vi "IQ Inversion.vi"(0 "input data":T1[](array[typedef])=[{"I"=0.0, "Q"=0.0, "overflow"=FALSE}, {"I"=0.0, "Q"=0.0, "overflow"=FALSE}, {"I"=0.0, "Q"=0.0, "overflow"=FALSE}, {"I"=0.0, "Q"=0.0, "overflow"=FALSE}, {"I"=0.0, "Q"=0.0, "overflow"=FALSE}, {"I"=0.0, "Q"=0.0, "overflow"=FALSE}, {"I"=0.0, "Q"=0.0, "overflow"=FALSE}, {"I"=0.0, "Q"=0.0, "overflow"=FALSE}, {"I"=0.0, "Q"=0.0, "overflow"=FALSE}, {"I"=0.0, "Q"=0.0, "overflow"=FALSE}, {"I"=0.0, "Q"=0.0, "overflow"=FALSE}, {"I"=0.0, "Q"=0.0, "overflow"=FALSE}, {"I"=0.0, "Q"=0.0, "overflow"=FALSE}, {"I"=0.0, "Q"=0.0, "overflow"=FALSE}, {"I"=0.0, "Q"=0.0, "overflow"=FALSE}, {"I"=0.0, "Q"=0.0, "overflow"=FALSE}], 5 "IQ inversion":cluster{"invert I":bool, "invert Q":bool}, 9 "input valid":bool=TRUE) -> (4 "output data":T1[](array[typedef]), 10 "output valid":bool)   [LabVIEW 2019]
uses:
  <instrlib>/_niInstr/DSP/v1/Shared/Public/IQ Data.ctl
  <instrlib>/_niInstr/DSP/v1/Shared/niInstr DSP v1 Shared.lvlib
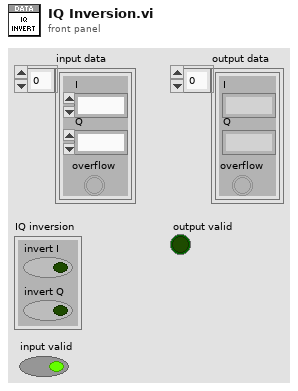
[diagram p1: front panel]
types:
  T1 = typedef "niInstr DSP v1 Shared.lvlib/IQ Data.ctl" = cluster{"I":fxp<+/-,18,1>, "Q":fxp<+/-,18,1>, "overflow":bool}
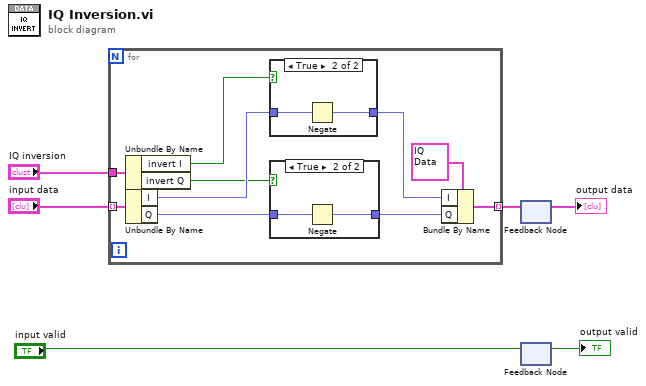
[diagram p0: block diagram]
diagram:
  n1 = for {
    tunnel: "input data" -> [w16] mode=indexing
    tunnel: "IQ inversion" -> [w15]
    tunnel: [w8] -> w4 mode=indexing
    n2 = Unbundle By Name(w15) -> ("invert I"=w14:bool, "invert Q"=w12:bool)
    n3 = Unbundle By Name(w16) -> ("I"=w13:fxp<+/-,18,1>, "Q"=w11:fxp<+/-,18,1>)
    n4 = case shown="True" w14 {
      tunnel: w13 -> [w20 w22]
      tunnel: [w20 w21] -> w10
      frame False {
      }
      frame True {
        n5 = Negate(x=w22) -> (-x=w21:fxp<+/-,18,1>)
      }
    }
    n6 = case shown="True" w12 {
      tunnel: w11 -> [w17 w19]
      tunnel: [w17 w18] -> w9
      frame False {
      }
      frame True {
        n7 = Negate(x=w19) -> (-x=w18:fxp<+/-,18,1>)
      }
    }
    n8 = Bundle By Name(cluster=T1 {"I"=0.0, "Q"=0.0, "overflow"=FALSE} ("data"), "I"=w10, "Q"=w9) -> (w8:T1)
  }
  n9 = feedback-in #1(w4) -> ()
  n10 = feedback #1() -> (→"output data":T1[])  [unwired: 1 in]
  n11 = feedback #2() -> (→"output valid":bool)  [unwired: 1 in]
  n12 = feedback-in #2("input valid") -> ()
